vi "ConvertPercentVbusToVoltage.vi"(11 "Vbus":dbl) -> (3 "Voltage":dbl)   [LabVIEW 2012]
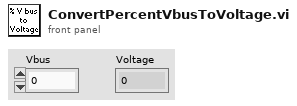
[diagram p1: front panel]
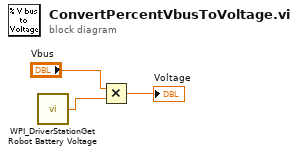
[diagram p0: block diagram]
diagram:
  n1 = call <vilib>:"WPI_DriverStationGet Robot Battery Voltage.vi"() -> ("robot battery voltage"=w3:dbl)  [unwired: 14 in, 1 out]
  n2 = Multiply(x="Vbus", y=w3) -> (x*y=→"Voltage":dbl)
